vi "OAT State Machine Detect Events.vi"   [LabVIEW 2017]
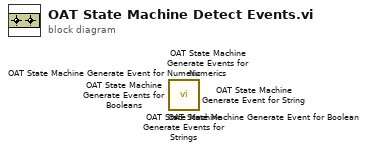
[diagram p0: block diagram]
diagram:
  n1 = call <vilib>:"OAT State Machine Generate Events for Strings.vi"() -> ()  [unwired: 8 in, 1 out]
  n2 = call <vilib>:"OAT State Machine Generate Events for Numerics.vi"() -> ()  [unwired: 8 in, 1 out]
  n3 = call <vilib>:"OAT State Machine Generate Events for Booleans.vi"() -> ()  [unwired: 8 in, 1 out]
  n4 = call <vilib>:"OAT State Machine Generate Event for String.vi"() -> ()  [unwired: 8 in, 1 out]
  n5 = call <vilib>:"OAT State Machine Generate Event for Numeric.vi"() -> ()  [unwired: 8 in, 1 out]
  n6 = call <vilib>:"OAT State Machine Generate Event for Boolean.vi"() -> ()  [unwired: 8 in, 1 out]
